vi "List People By Role.vi"(8 "error in (no error)":errorcluster, 10 "Roles":T1, 11 "Coffee Shop In":refnum<class "Coffee Shop.lvclass">) -> (0 "error out":errorcluster, 2 "Names":string[](array[string]), 3 "Coffee Shop Out":refnum<class "Coffee Shop.lvclass">)   [LabVIEW 2020, in "Coffee Shop.lvclass"]
uses:
  Coffee Shop.lvclass
  C:/Program Files (x86)/National Instruments/LabVIEW 2020/vi.lib/Asteme/Triarc Framework/Process/Process.lvclass
  Public/Roles.ctl
  <vilib>/Asteme/Triarc Framework/Process/Process.lvclass/Process.ctl
  <vilib>/Asteme/Triarc Framework/Process/Public/Lifecycle/Get Lifecycle State.vi
  <vilib>/Asteme/Triarc Framework/Process/Private/SubVIs/Enqueue Request Message.vi
  <vilib>/Utility/error.llb/Clear Errors.vi
  <vilib>/AdvancedString/1D String Array to Delimited String.vi
  <vilib>/Utility/error.llb/Error Cluster From Error Code.vi
  <vilib>/Asteme/Triarc Framework/Process/Private/SubVIs/Wait for Response Message.vi
  <vilib>/Asteme/Triarc Framework/Process/Process.lvclass
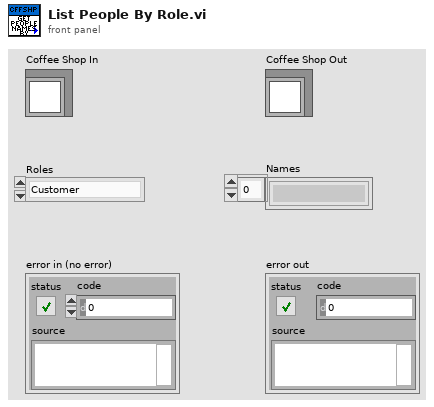
[diagram p1: front panel]
types:
  T1 = typedef "Coffee Shop.lvclass/Roles.ctl" = enum16{"Customer", "Barista", "Cashier"}
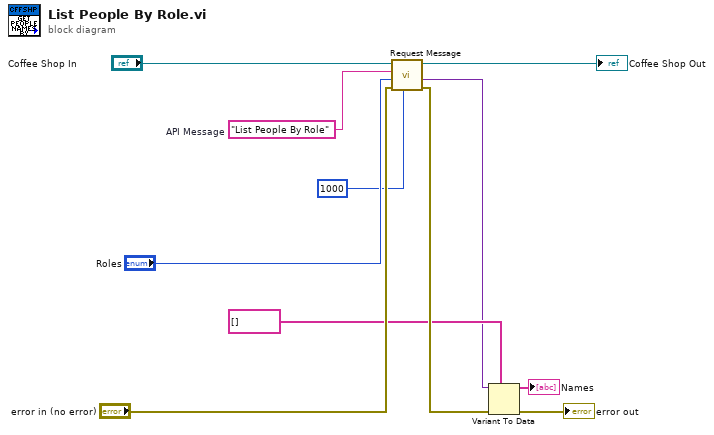
[diagram p0: block diagram]
diagram:
  w8 = "List People By Role"  # API Message
  n1 = call <vilib>:"Request Message.vi"("timeout in ms (-1)"=1000, "error in (no error)"="error in (no error)", "Request Message Data"="Roles", "Request Message"=w8, "Process In"="Coffee Shop In") -> ("error out"=w10:errorcluster, "Response Message Data"=w3:variant, "Process Out"=→"Coffee Shop Out":refnum<class "Coffee Shop.lvclass">)  [unwired: 2 in, 2 out]
  n2 = Variant To Data(error in=w10, type=string[] [], Variant=w3) -> (data=→"Names":string[], error out=→"error out":errorcluster)
